vi "Exemple1.vi"() -> ()   [LabVIEW 2018]
panel:
  in  "a":dbl
  out "c":dbl
  in  "b":dbl
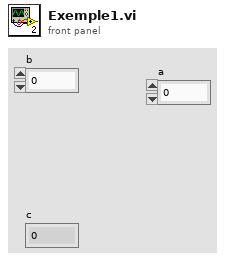
[diagram p1: front panel]
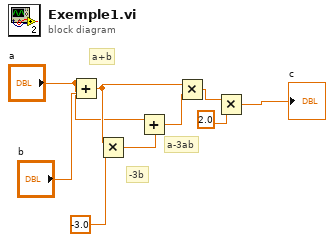
[diagram p0: block diagram]
diagram:
  # "a-3ab"
  # "-3b"
  # "a+b"
  n1 = Add(x="a", y="b") -> (x+y=w3:dbl)
  n2 = Multiply(x=w3, y=-3.0 ("b")) -> (x*y=w5:dbl)
  n3 = Add(x="a", y=w5) -> (x+y=w4:dbl)
  n4 = Multiply(x=w3, y=w4) -> (x*y=w8:dbl)
  n5 = Multiply(x=w8, y=2.0 ("c")) -> (x*y=→"c":dbl)
